vi "Stitching-Get experiment folder name string.vi"(10 "folder names":string[](array[string])=["141120_14_28_12", "141120_14_28_14", "141120_14_28"], 11 "Experiment folder user string":string="141120_14_28_14 asdfsg") -> (3 "Actual experiment folder name":string)   [LabVIEW 2013]
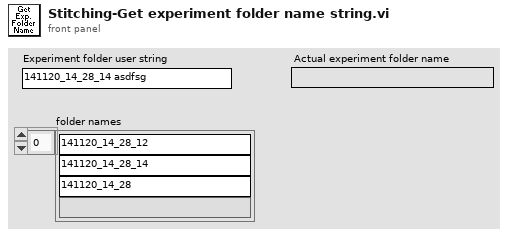
[diagram p1: front panel]
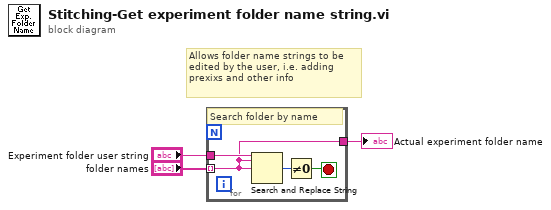
[diagram p0: block diagram]
diagram:
  # "Allows folder name strings to be edited by the user, i.e. adding prexixs and other info"
  n1 = for {
    tunnel: "folder names" -> [w4] mode=indexing
    tunnel: "Experiment folder user string" -> [w5]
    tunnel: [w4] -> w3
    stop <- w6 stop-if-true
    # "Search folder by name"
    n2 = Search and Replace String(input string=w5, search string=w4, replace string=w4) -> (number of replacements=w7:i32)  [unwired: 5 in, 3 out]
    n3 = Not Equal To 0?(x=w7) -> (x != 0?=w6:bool)
  }
  "Actual experiment folder name" <- w3
